vi "Read Float timed.vi"(4 "delay before write":u32=400, 6 "Parity":u16(ring)=2 items=["None", "Odd", "Even", "Mark", "Space"], 8 "error in":errorcluster, 9 "State":i16, 10 "Time":dbl format="%.2f", 11 "set point inputs":T3) -> (0 "error out":errorcluster, 1 "output value":dbl, 2 "read":bool, 3 "VISA resource name out":refnum<visa-resource-name>)   [LabVIEW 2019]
panel:
  in  "register":T1
  out "register array":T2(array[cluster])
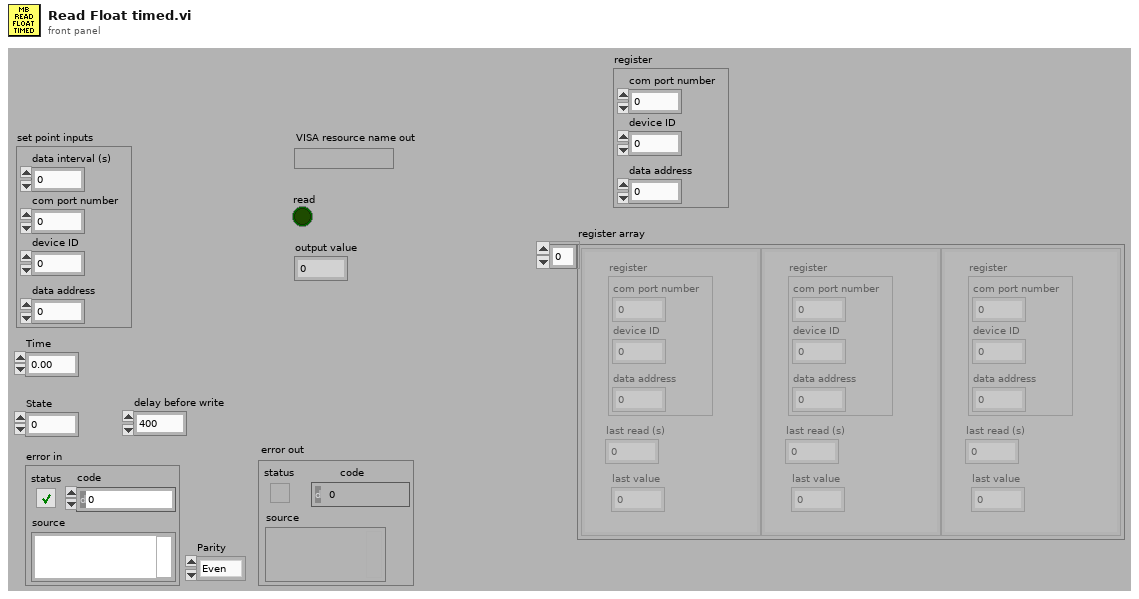
[diagram p1: front panel]
types:
  T1 = cluster{"com port number":u8, "device ID":u8, "data address":u8}
  T2 = cluster{"register":cluster{"com port number":u8, "device ID":u8, "data address":u8}, "last read (s)":dbl, "last value":dbl}[]
  T3 = cluster{"data interval (s)":dbl, "com port number":u8, "device ID":u8, "data address":u8}
  T4 = cluster{"register":cluster{"com port number":u8, "device ID":u8, "data address":u8}, "last read (s)":dbl, "last value":dbl}
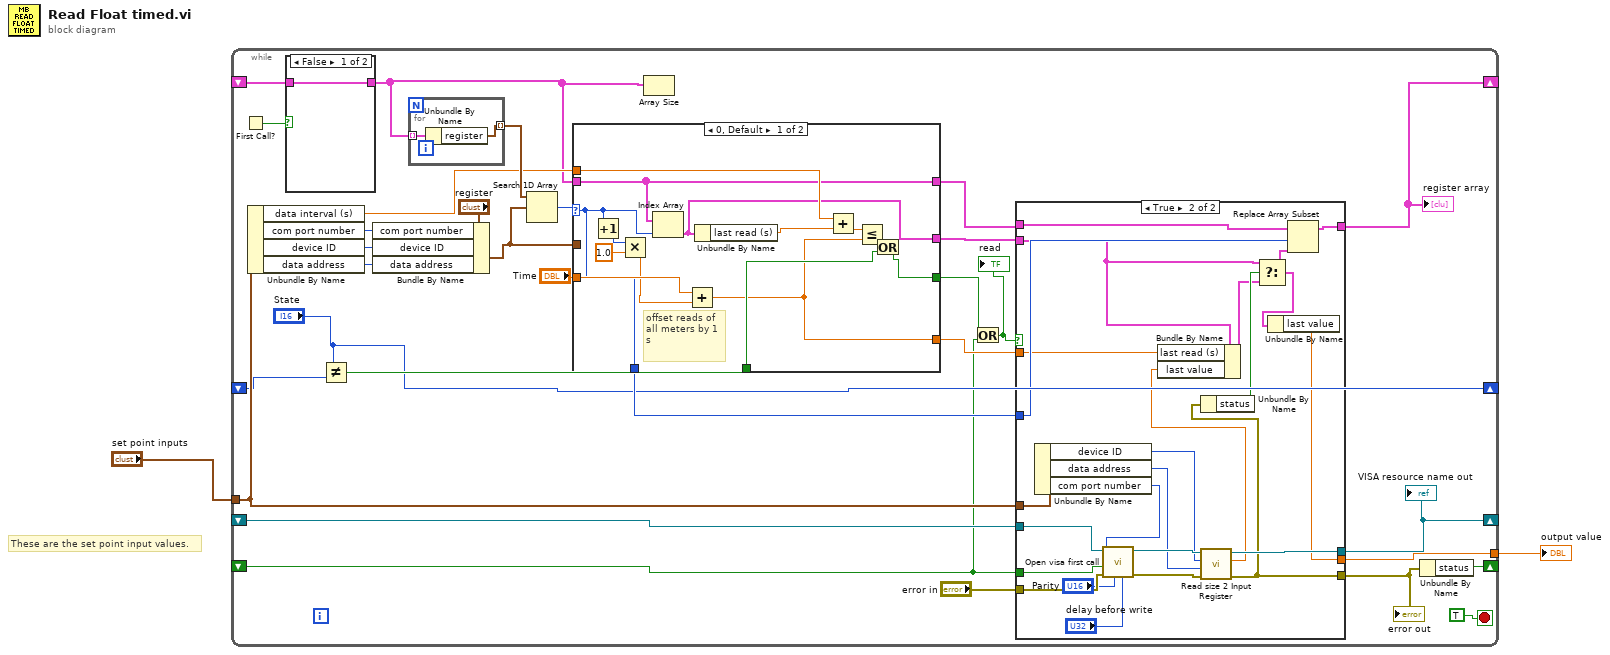
[diagram p0: block diagram]
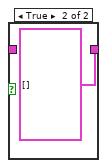
[diagram p2: hidden frame]
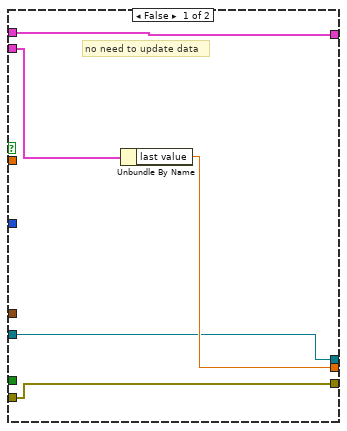
[diagram p3: hidden frame]
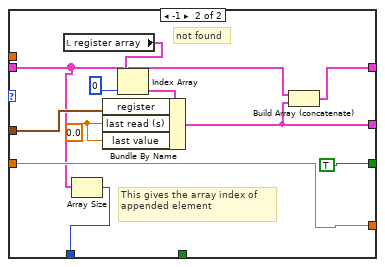
[diagram p4: hidden frame]
diagram:
  # "These are the set point input values."
  n1 = while {
    tunnel: [w28] -> w2
    shift-right: [w30] -> _
    shift-left: _ -> [w32]
    tunnel: "set point inputs" -> [w26]
    shift-right: [w31] -> _
    shift-left: _ -> [w5]
    shift-right: [w16] -> _
    shift-left: _ -> [w8]
    shift-right: ["State"] -> _
    shift-left: _ -> [w10]
    stop <- TRUE stop-if-true
    n2 = First Call?() -> (First Call?: T/F=w9:bool)
    n3 = Unbundle By Name(w26) -> ("data interval (s)"=w19:dbl, "com port number"=w24:u8, "device ID"=w23:u8, "data address"=w22:u8)
    n4 = case shown="False" w9 {
      tunnel: w8 -> [w34 _]
      tunnel: [w34 T2 []] -> w3
      frame False {
      }
      frame True {
      }
    }
    n5 = Not Equal?(x="State", y=w10) -> (x != y?=w18:bool)
    n6 = Bundle By Name(cluster="register", "com port number"=w24, "device ID"=w23, "data address"=w22) -> (w25:T1)
    n7 = for {
      tunnel: w3 -> [w37] mode=indexing
      tunnel: [w36] -> w20 mode=indexing
      n8 = Unbundle By Name(w37) -> ("register"=w36:T1)
    }
    n9 = Search 1D Array(1D array=w20, element=w25) -> (index of element=w27:i32)  [unwired: 1 in]
    n10 = case shown="0, Default" w27 {
      selector: w27 -> [w66 _]
      tunnel: [w74 TRUE] -> w6
      tunnel: w3 -> [w73 w81]
      tunnel: w25 -> [_ w88]
      tunnel: [w73 w89] -> w17
      tunnel: w19 -> [w79 _]
      tunnel: w18 -> [w75 _]
      tunnel: [w66 w80] -> w15
      tunnel: [w70 w82] -> w14
      tunnel: [w72 w84] -> w13
      tunnel: "Time" -> [w71 w82]
      frame 0, Default {
        # "offset reads of all meters by 1 s"
        n11 = Increment(x=w66) -> (x+1=w67:i32)
        n12 = Multiply(x=w67, y=sgl 1.0) -> (x*y=w69:sgl)
        n13 = Index Array(array=w73, index=w66) -> (element=w72:T4)
        n14 = Add(x=w71, y=w69) -> (x+y=w70:dbl)
        n15 = Unbundle By Name(w72) -> ("last read (s)"=w78:dbl)
        n16 = Add(x=w79, y=w78) -> (x+y=w77:dbl)
        n17 = Less Or Equal?(x=w77, y=w70) -> (x <= y?=w76:bool)
        n18 = Or(x=w76, y=w75) -> (x .or. y?=w74:bool)
      }
      frame -1 {
        w83 = 0.0
        # "This gives the array index of appended element"
        # "not found"
        n19 = local read "register array"() -> (w85:T2)
        n20 = Array Size(array=w81) -> (size(s)=w80:i32)
        n21 = Index Array(array=w85, index=0) -> (element=w87:T4)
        n22 = Bundle By Name(cluster=w87, "register"=w88, "last read (s)"=w83, "last value"=w83) -> (w84:T4)
        n23 = Build Array (concatenate)(w81, w84) -> (w89:T2)
      }
    }
    n24 = Array Size(array=w3) -> ()  [unwired: 1 out]
    n25 = Or(x=w6, y=w5) -> (x .or. y?=w4:bool)
    "read" <- w4
    n26 = case shown="True" w4 {
      tunnel: w32 -> [w39 w65]
      tunnel: w5 -> [_ w50]
      tunnel: [w39 w64] -> w30
      tunnel: [w38 w49] -> w29
      tunnel: [w40 w44] -> w28
      tunnel: w26 -> [_ w60]
      tunnel: w17 -> [w42 w58]
      tunnel: [w42 w57] -> w16
      tunnel: w15 -> [_ w59]
      tunnel: w14 -> [_ w55]
      tunnel: w13 -> [w41 w46]
      tunnel: "error in" -> [w38 w54]
      frame False {
        # "no need to update data"
        n27 = Unbundle By Name(w41) -> ("last value"=w40:dbl)
      }
      frame True {
        n28 = Unbundle By Name(w60) -> ("device ID"=w61:u8, "data address"=w53:u8, "com port number"=w51:u8)
        n29 = call "Open visa first call.vi"("delay before write"="delay before write", "Parity"="Parity", "error in (no error)"=w54, "error"=w50, "Com port"=w51, "VISA Refnum in"=w65) -> ("error out"=w62:errorcluster, "VISA Refnum out"=w63:refnum<visa-resource-name>)  [unwired: 4 in]
        n30 = call "Read size 2 Input Register.vi"("error in"=w62, "data address"=w53, "device ID"=w61, "VISA resource name"=w63) -> ("error out"=w49:errorcluster, "Meter reading"=w56:sgl, "VISA resource name out"=w64:refnum<visa-resource-name>)  [unwired: 3 in, 2 out]
        n31 = Bundle By Name(cluster=w46, "last read (s)"=w55, "last value"=w56) -> (w47:T4)
        n32 = Unbundle By Name(w49) -> ("status"=w48:bool)
        n33 = Select(t=w46, s=w48, f=w47) -> (s? t:f=w45:T4)
        n34 = Unbundle By Name(w45) -> ("last value"=w44:dbl)
        n35 = Replace Array Subset(array=w58, new element=w45, index=w59) -> (w57:T2)
      }
    }
    "VISA resource name out" <- w30
    "error out" <- w29
    "register array" <- w16
    n36 = Unbundle By Name(w29) -> ("status"=w31:bool)
  }
  "output value" <- w2
